vi "XIPIN_JESD204_PHY_3_0.vi"   [LabVIEW 2017]
doc: "The Xilinx JESD204 PHY core implements a Physical Layer interface to simplify the instantiation of the GTXE2, GTHE2, GTPE2, GTHE3 and GTYE3 transceivers when used with the JESD204 core.\n------------------------------------\n<b>Need License</b> : No\n<b>Interface</b> : AXI4"
uses:
  <vilib>/rvi/XilinxIP/XIPIN_XNode/niFpgaXIPIN.xnode
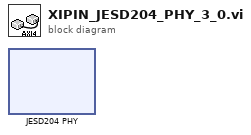
[diagram p0: block diagram]
diagram:
  n1 = xnode ("JESD204 PHY")() -> ()
